vi "Panel.vi"(11 "Terminal in":refnum<class "Terminal.lvclass">) -> ()   [LabVIEW 2020, in "PicoG-Processor.lvlib" / "Terminal.lvclass"]
uses:
  Terminal.lvclass
panel:
  in  "Content":string
  in  "Device List":i32(listbox)
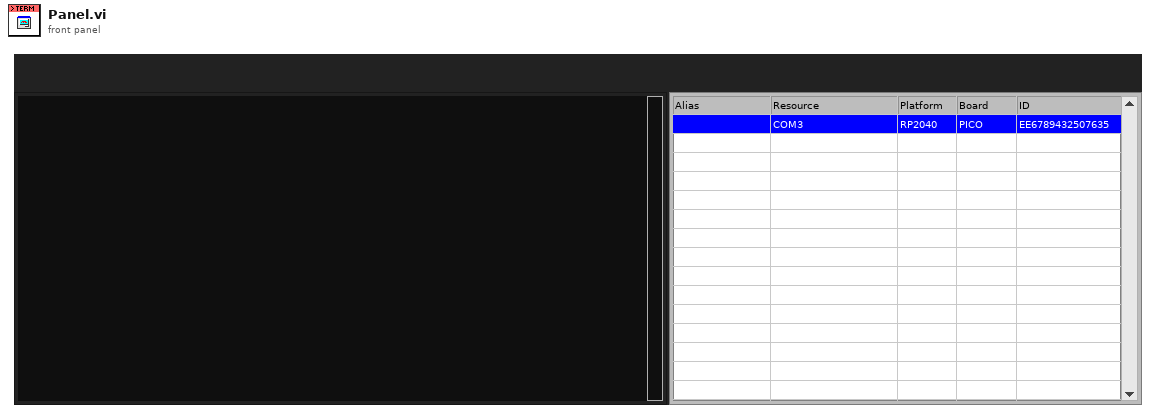
[diagram p1: front panel]
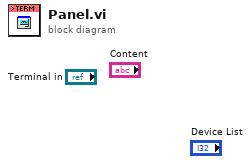
[diagram p0: block diagram]
diagram:
